vi "压缩感知重建方法.vi"(0 "模块选择簇":T3, 5 "光源散斑簇":T2, 7 "图像信息簇":T1, 9 "散斑图像作用结果":dbl[][](array[numeric])) -> (4 "未归一化图像二维数组":i32[][](array[numeric]))   [LabVIEW 2018]
uses:
  <vilib>/Analysis/baseanly.llb/Mean (DBL).vi
  <vilib>/Analysis/2dsp.llb/2D Inverse DCT.vi
  <vilib>/Analysis/NI_AALPro.lvlib
  <vilib>/Analysis/NI_AALBase.lvlib
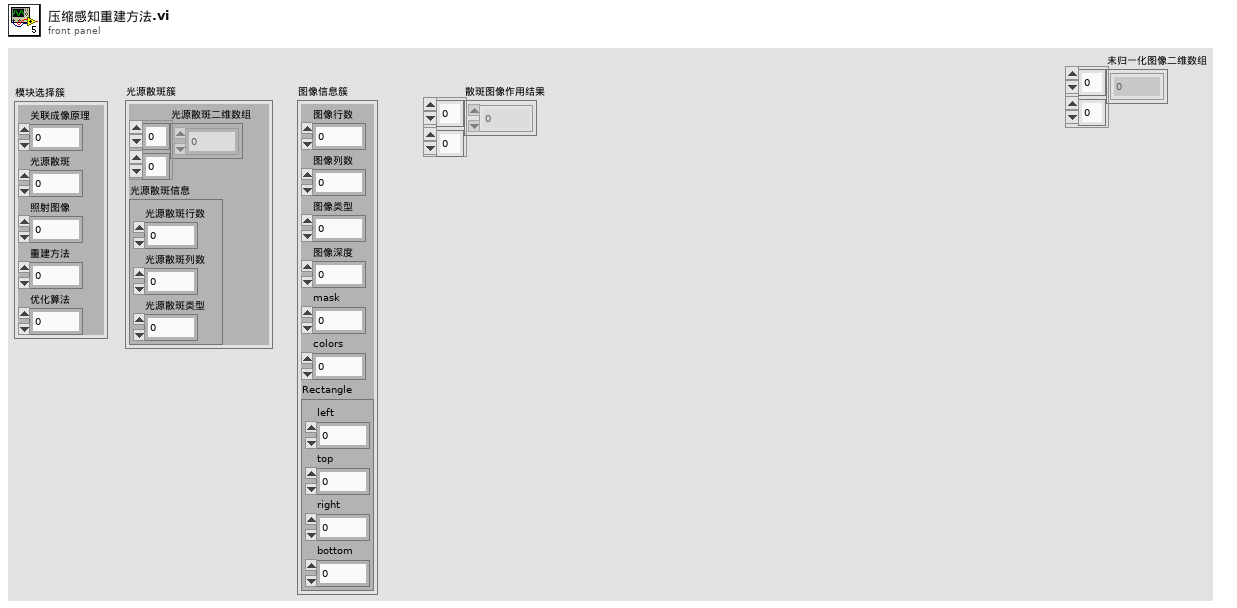
[diagram p1: front panel]
types:
  T1 = cluster{"图像行数":dbl, "图像列数":dbl, "图像类型":dbl, "图像深度":i32, "mask":i32, "colors":i32, "Rectangle":cluster{"left":i16, "top":i16, "right":i16, "bottom":i16}}
  T2 = cluster{"光源散斑二维数组":dbl[][], "光源散斑信息":cluster{"光源散斑行数":dbl, "光源散斑列数":dbl, "光源散斑类型":dbl}}
  T3 = cluster{"关联成像原理":i32, "光源散斑":i32, "照射图像":i32, "重建方法":i32, "优化算法":i32}
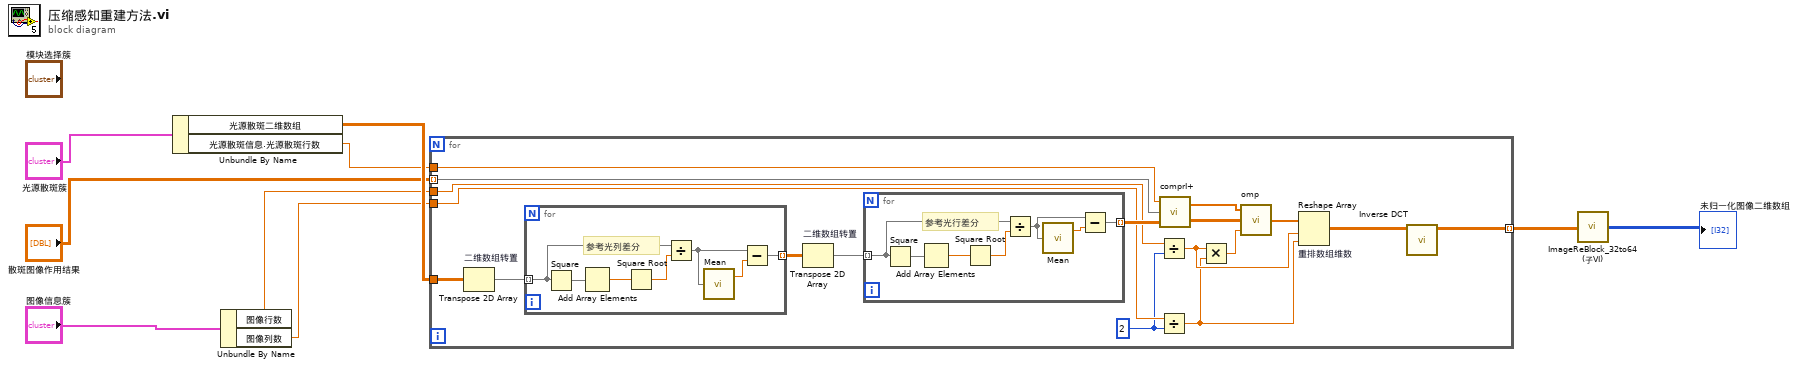
[diagram p0: block diagram]
diagram:
  n1 = Unbundle By Name("光源散斑簇") -> ("光源散斑二维数组"=w9:dbl[][], "光源散斑信息.光源散斑行数"=w8:dbl)
  n2 = Unbundle By Name("图像信息簇") -> ("图像行数"=w2:dbl, "图像列数"=w1:dbl)
  n3 = for {
    tunnel: w9 -> [w27]
    tunnel: "散斑图像作用结果" -> [w26] mode=indexing
    tunnel: w8 -> [w25]
    tunnel: [w17] -> w6 mode=indexing
    tunnel: w2 -> [w15]
    tunnel: w1 -> [w14]
    w13 = 2
    n4 = Transpose 2D Array "二维数组转置"(2D array=w27) -> (transposed array=w24:dbl[][])
    n5 = for {
      tunnel: w24 -> [w35] mode=indexing
      tunnel: [w36] -> w21 mode=indexing
      # "参考光列差分"
      n6 = Square(x=w35) -> (x^2=w40:dbl[])
      n7 = Add Array Elements(numeric array=w40) -> (sum=w39:dbl)
      n8 = Square Root(x=w39) -> (sqrt(x)=w38:dbl)
      n9 = Divide(x=w35, y=w38) -> (x/y=w37:dbl[])
      n10 = call-poly <vilib>:"Mean.vi"("X"=w37) -> ("mean"=w41:dbl)  [unwired: 1 out]
      n11 = Subtract ("Subtract.vi")(x=w37, y=w41) -> (x-y=w36:dbl[])
    }
    n12 = Transpose 2D Array "二维数组转置"(2D array=w21) -> (transposed array=w20:dbl[][])
    n13 = for {
      tunnel: w20 -> [w30] mode=indexing
      tunnel: [w28] -> w16 mode=indexing
      # "参考光行差分"
      n14 = Square(x=w30) -> (x^2=w33:dbl[])
      n15 = Add Array Elements(numeric array=w33) -> (sum=w32:dbl)
      n16 = Square Root(x=w32) -> (sqrt(x)=w31:dbl)
      n17 = Divide(x=w30, y=w31) -> (x/y=w29:dbl[])
      n18 = call-poly <vilib>:"Mean.vi"("X"=w29) -> ("mean"=w34:dbl)  [unwired: 1 out]
      n19 = Subtract ("Subtract.vi")(x=w29, y=w34) -> (x-y=w28:dbl[])
    }
    n20 = Divide(x=w15, y=w13) -> (x/y=w12:dbl)
    n21 = Divide(x=w14, y=w13) -> (x/y=w11:dbl)
    n22 = call "comprI+.vi"("I"=w16, "B"=w26, "采样点数"=w25) -> ("I+"=w23:dbl[][], "B+"=w22:dbl[])
    n23 = Multiply(x=w12, y=w11) -> (x*y=w10:dbl)
    n24 = call "omp.vi"("N"=w10, "T"=w23, "s"=w22) -> ("hat_y"=w19:dbl[])
    n25 = Reshape Array "重排数组维数"(w19, w12, w11) -> (w18:dbl[][])
    n26 = call-poly <vilib>:"Inverse DCT.vi"("DCT {X}"=w18) -> ("X"=w17:dbl[][])  [unwired: 10 out]
  }
  n27 = call "ImageReBlock_32to64 (子VI).vi"("BlockImg"=w6) -> ("ReBlockImg"=→"未归一化图像二维数组":i32[][])
